vi "add channel to configuration.vi"(8 "error in":errorcluster, 10 "TBM channel in":refnum<class "EIP Tags Channel.lvclass">, 11 "EthernetIP configuration in":refnum<class "EIP Tags Configuration.lvclass">) -> (0 "error out":errorcluster, 3 "EthernetIP configuration out":refnum<class "EIP Tags Configuration.lvclass">)   [LabVIEW 2013, in "EIP Tags Configuration.lvclass"]
uses:
  EIP Tags Configuration.lvclass
  channel/EIP Tags Channel.lvclass
  <vilib>/NI/Tag Bus/tag/tag descriptor.lvclass/tag descriptor.ctl
  <vilib>/NI/Tag Bus/tag/Data Type.ctl
  channel/EIP Tags Channel.lvclass/EIP Tags Channel.ctl
  EIP Tags Configuration.lvclass/EIP Tags Configuration.ctl
  channel/Read EIP Tag UUID.vi
  channel/Read element.vi
  <vilib>/NI/Tag Bus/tag/read data type.vi
  <vilib>/NI/Tag Bus/tag/tag descriptor.lvclass
  <vilib>/NI/Configuration Framework/NISE_CEF_TreeControl.lvlib
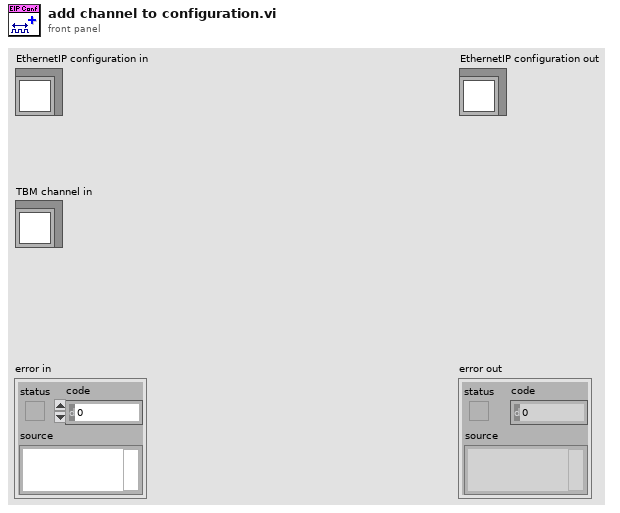
[diagram p1: front panel]
types:
  T1 = typedef "tag bus.lvlib/tag descriptor.lvclass/Data Type.ctl" = enum16{"Double", "Single", "I64", "I32", "I16", "I8", "U64", "U32", "U16", "U8", "Boolean", "String", "Array of Double", "Array of Single", "Array of I64", "Array of I32", "Array of I16", "Array of I8", "Array of U64", "Array of U32", "Array of U16", "Array of U8", "Array of Boolean", "Array of String"}
  T2 = typedef "EIP Tags Configuration.lvclass/eip tag definition.ctl" = cluster{"eip tag types":T3, "unique tag name":string, "Number of Elements":u32}
  T3 = typedef "EIP Tags Configuration.lvclass/eip tag types.ctl" = enum16{"SINT", "INT", "DINT", "REAL", "BOOL", "STRING"}
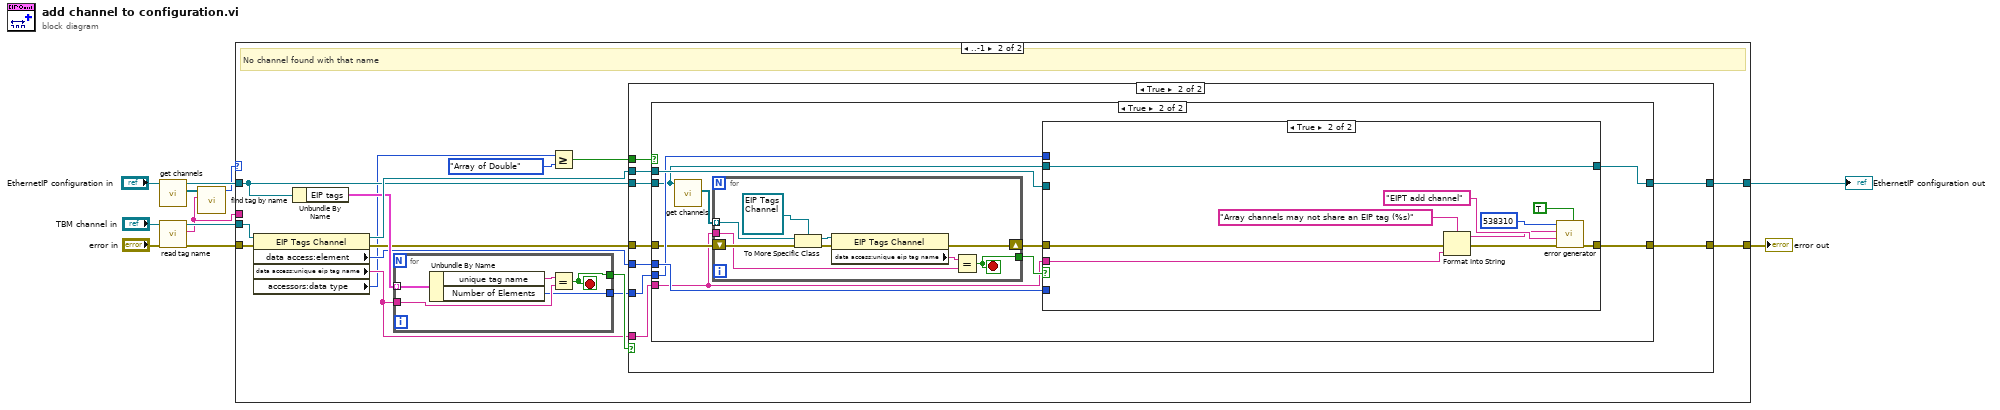
[diagram p0: block diagram]
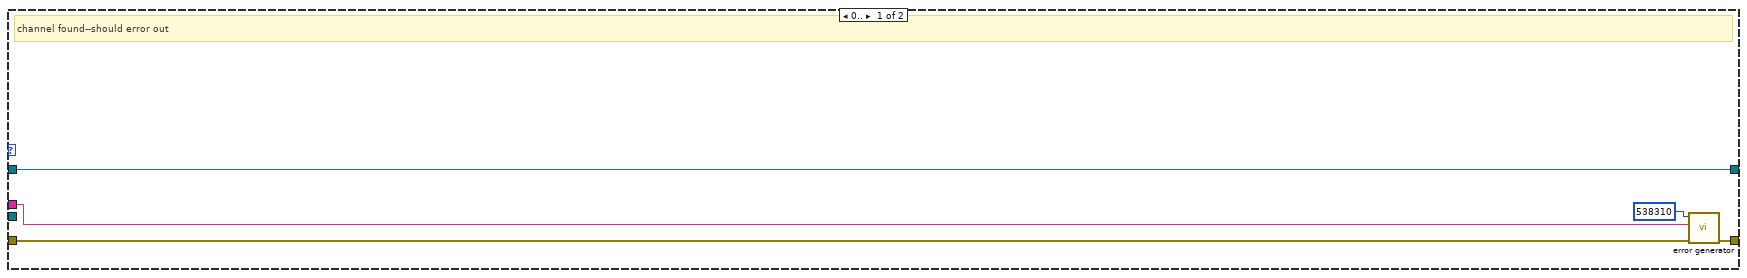
[diagram p2: hidden frame]
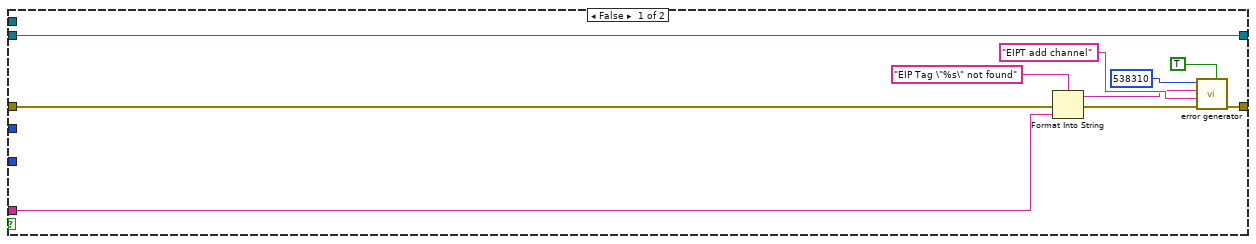
[diagram p3: hidden frame]
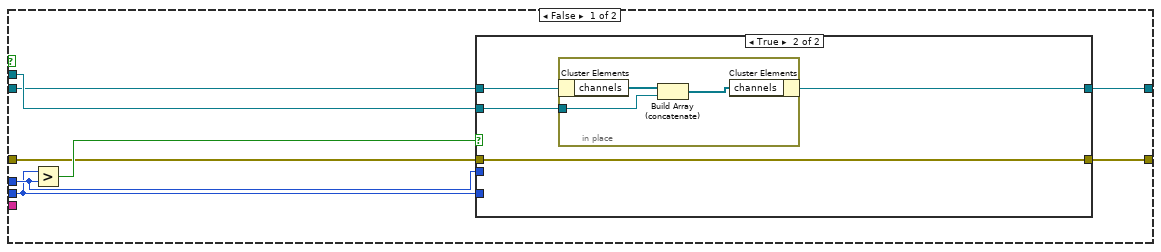
[diagram p4: hidden frame]
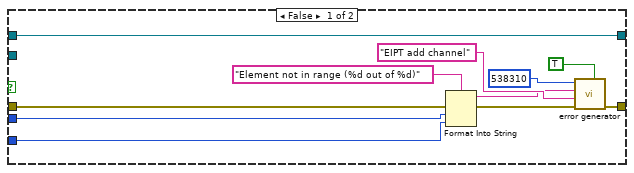
[diagram p5: hidden frame]
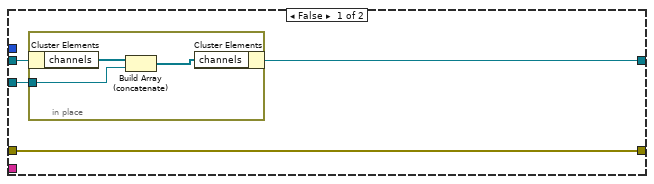
[diagram p6: hidden frame]
diagram:
  n1 = call-dynamic "get channels.vi"("EthernetIP configuration in"="EthernetIP configuration in") -> ("channels"=w5:refnum<class "TBM channel.lvclass">[], "EthernetIP configuration out"=w11:refnum<class "EIP Tags Configuration.lvclass">)  [unwired: 9 in]
  n2 = call <vilib>:"read tag name.vi"("error in"="error in", "system tag in"="TBM channel in") -> ("error out"=w2:errorcluster, "name"=w3:string, "system tag out"=w10:refnum<class "EIP Tags Channel.lvclass">)  [unwired: 7 in]
  n3 = call <vilib>:"find tag by name.vi"("name"=w3, "tags in"=w5) -> ("index"=w4:i32)  [unwired: 9 in]
  n4 = case shown="..-1" w4 {
    tunnel: [w16 w23] -> w8
    tunnel: w3 -> [w14 _]
    tunnel: w2 -> [w13 w31]
    tunnel: w11 -> [w12 w27]
    tunnel: w10 -> [_ w29]
    tunnel: [w12 w30] -> w7
    frame 0.. {
      # "channel found--should error out"
      n5 = call <vilib>:"error generator.vi"("error in"=w13, "append error message"=w14, "error code (0)"=538310) -> ("error out"=w16:errorcluster)  [unwired: 6 in]
    }
    frame ..-1 {
      # "No channel found with that name"
      n6 = property class="EIP Tags Channel"(reference=w29, error in=w31) -> (reference out=w28:refnum<class "EIP Tags Channel.lvclass">, error out=w24:errorcluster, "data access:element"=w20:i32, "data access:unique eip tag name"=w22:string, "accessors:data type"=w19:T1)
      n7 = Unbundle By Name(w27) -> ("EIP tags"=w26:T2[])
      n8 = for {
        tunnel: w26 -> [w118] mode=indexing
        tunnel: w22 -> [w117]
        tunnel: [w116] -> w21
        tunnel: [w115] -> w25
        stop <- w115 stop-if-true
        n9 = Unbundle By Name(w118) -> ("unique tag name"=w114:string, "Number of Elements"=w116:u32)
        n10 = Equal?(x=w114, y=w117) -> (x = y?=w115:bool)
      }
      n11 = Greater Or Equal?(x=w19, y=Data_Type."Array of Double") -> (x >= y?=w17:bool)
      n12 = case shown="True" w25 {
        tunnel: [w41 w50] -> w30
        tunnel: w28 -> [_ w49]
        tunnel: w27 -> [w41 w48]
        tunnel: w24 -> [w38 w47]
        tunnel: [w39 w46] -> w23
        tunnel: w22 -> [w33 w42]
        tunnel: w21 -> [_ w44]
        tunnel: w20 -> [_ w45]
        tunnel: w17 -> [_ w43]
        frame False {
          n13 = Format Into String(format string="EIP Tag \"%s\" not found", error in=w38, w33) -> (resulting string=w34:string, error out=w35:errorcluster)  [unwired: 1 in]
          n14 = call <vilib>:"error generator.vi"("concatenate (F)"=TRUE, "error in"=w35, "source"="EIPT add channel", "append error message"=w34, "error code (0)"=538310) -> ("error out"=w39:errorcluster)  [unwired: 4 in]
        }
        frame True {
          n15 = case shown="True" w43 {
            tunnel: [w58 w87] -> w50
            tunnel: w49 -> [w57 w86]
            tunnel: w48 -> [w56 w82]
            tunnel: w47 -> [w54 w80]
            tunnel: [w53 w85] -> w46
            tunnel: w45 -> [w52 w84]
            tunnel: w44 -> [w51 w83]
            tunnel: w42 -> [_ w77]
            frame False {
              n16 = Greater?(x=w51, y=w52) -> (0:w55:bool)
              n17 = case shown="True" w55 {
                tunnel: [w69 w73] -> w58
                tunnel: w57 -> [_ w72]
                tunnel: w56 -> [w69 w71]
                tunnel: w54 -> [w62 w70]
                tunnel: [w61 w70] -> w53
                tunnel: w52 -> [w60 _]
                tunnel: w51 -> [w59 _]
                frame False {
                  n18 = Format Into String(format string="Element not in range (%d out of %d)", error in=w62, w60, w59) -> (resulting string=w64:string, error out=w65:errorcluster)  [unwired: 1 in]
                  n19 = call <vilib>:"error generator.vi"("concatenate (F)"=TRUE, "error in"=w65, "source"="EIPT add channel", "append error message"=w64, "error code (0)"=538310) -> ("error out"=w61:errorcluster)  [unwired: 4 in]
                }
                frame True {
                  n20 = in-place {
                    in-place-border: w72 -> [w76]
                    n21 = in-place-cluster #1(w71) -> ("channels"=w74:refnum<class "EIP Tags Channel.lvclass">[])
                    n22 = Build Array (concatenate)(w74, w76) -> (w75:refnum<class "EIP Tags Channel.lvclass">[])
                    n23 = in-place-cluster #1("channels"=w75) -> (w73:refnum<class "EIP Tags Configuration.lvclass">)
                  }
                }
              }
            }
            frame True {
              n24 = call-dynamic "get channels.vi"("EthernetIP configuration in"=w82) -> ("channels"=w81:refnum<class "TBM channel.lvclass">[])  [unwired: 9 in, 1 out]
              n25 = for {
                tunnel: w81 -> [w96] mode=indexing
                shift-right: [w93] -> w79
                shift-left: w80 -> [w92]
                tunnel: w77 -> [w89]
                tunnel: [w88] -> w78
                stop <- w88 stop-if-true
                n26 = To More Specific Class(target class=refnum<class "EIP Tags Channel.lvclass"> refnum ("TBM channel in 2"), reference=w96, error in=w92) -> (specific class reference=w95:refnum<class "EIP Tags Channel.lvclass">, error out=w94:errorcluster)
                n27 = property class="EIP Tags Channel"(reference=w95, error in=w94) -> (error out=w93:errorcluster, "data access:unique eip tag name"=w90:string)  [unwired: 1 out]
                n28 = Equal?(x=w90, y=w89) -> (x = y?=w88:bool)
              }
              n29 = case shown="True" w78 {
                tunnel: [w100 w113] -> w87
                tunnel: w86 -> [w99 _]
                tunnel: w82 -> [w98 w113]
                tunnel: w79 -> [w97 w106]
                tunnel: [w97 w105] -> w85
                tunnel: w84 -> [_ _]
                tunnel: w83 -> [_ _]
                tunnel: w77 -> [_ w104]
                frame False {
                  n30 = in-place {
                    in-place-border: w99 -> [w103]
                    n31 = in-place-cluster #2(w98) -> ("channels"=w101:refnum<class "EIP Tags Channel.lvclass">[])
                    n32 = Build Array (concatenate)(w101, w103) -> (w102:refnum<class "EIP Tags Channel.lvclass">[])
                    n33 = in-place-cluster #2("channels"=w102) -> (w100:refnum<class "EIP Tags Configuration.lvclass">)
                  }
                }
                frame True {
                  n34 = Format Into String(format string="Array channels may not share an EIP tag (%s)", error in=w106, w104) -> (resulting string=w108:string, error out=w109:errorcluster)  [unwired: 1 in]
                  n35 = call <vilib>:"error generator.vi"("concatenate (F)"=TRUE, "error in"=w109, "source"="EIPT add channel", "append error message"=w108, "error code (0)"=538310) -> ("error out"=w105:errorcluster)  [unwired: 4 in]
                }
              }
            }
          }
        }
      }
    }
  }
  "error out" <- w8
  "EthernetIP configuration out" <- w7
